vi "Set Filter Parameters.vi"(5 "noise":i32, 6 "smooth":i32, 7 "accept":sgl, 8 "error in (no error)":errorcluster, 9 "range":i32, 10 "sensitivity":sgl, 11 "width":i32) -> (0 "error out":errorcluster, 3 "function return":u32)   [LabVIEW 2014, in "atmcd32d.lvlib"]
doc: "unsigned int WINAPI SetFilterParameters(int width, float sensitivity, int range, float accept, int smooth, int noise);"
uses:
  atmcd32d.lvlib
  atmcd32d.dll
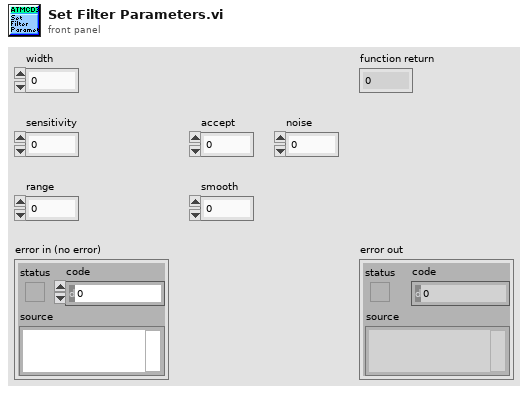
[diagram p1: front panel]
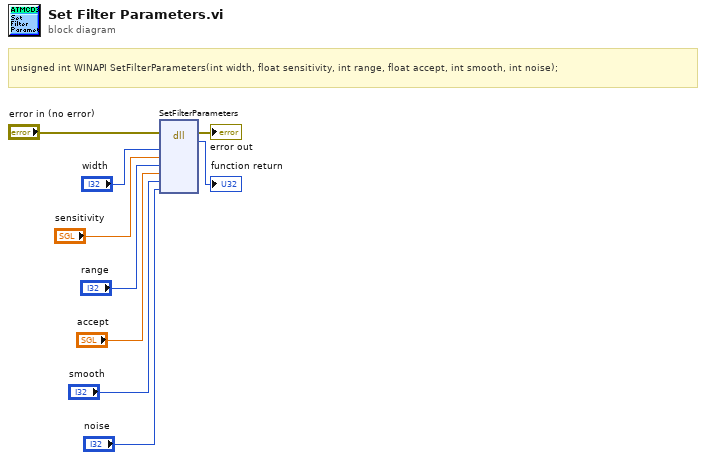
[diagram p0: block diagram]
diagram:
  # "unsigned int WINAPI SetFilterParameters(int width, float sensitivity, int range, float accept, int smooth, int noise);"
  n1 = dll-call lib="C:/Users/Bakir/Documents/Lambda2-Testing/lib/Andorlib/atmcd32d.*" fn="SetFilterParameters"(error in="error in (no error)", "width"="width", "sensitivity"="sensitivity", "range"="range", "accept"="accept", "smooth"="smooth", "noise"="noise") -> (error out=→"error out":errorcluster, →"function return":u32)  [unwired: 8 in, 1 out]
